vi "HaltDev.vi"(0 "输入簇":T1) -> ()   [LabVIEW 2012]
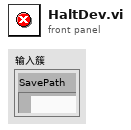
[diagram p1: front panel]
types:
  T1 = cluster{"SavePath":path, "SAVE?":bool, "connection ID":refnum<k5>}
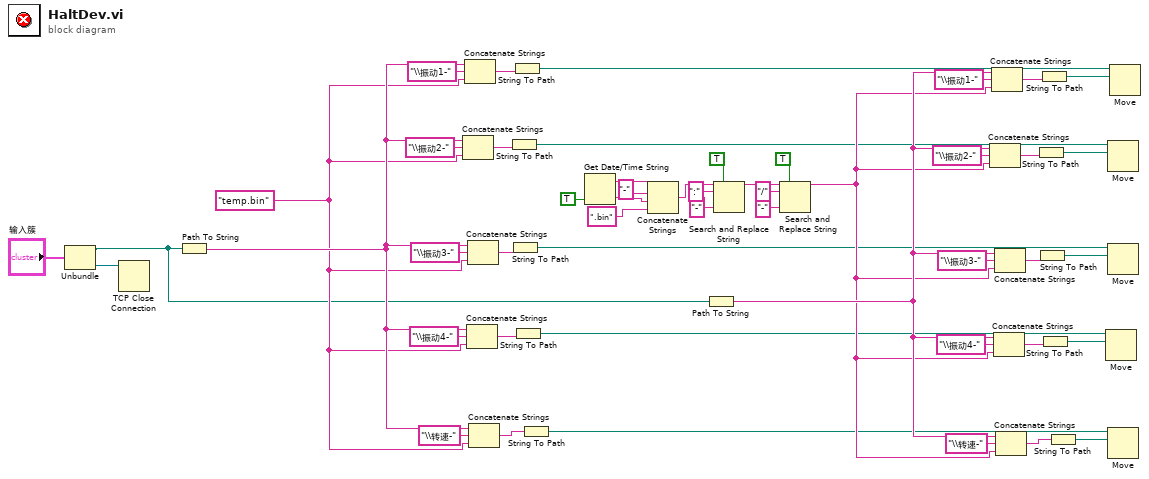
[diagram p0: block diagram]
diagram:
  w14 = "temp.bin" ("字符串")
  n1 = Unbundle("输入簇") -> ("SavePath"=w2:path, "connection ID"=w1:refnum<k5>)  [unwired: 1 out]
  n2 = TCP Close Connection(connection ID=w1) -> ()  [unwired: 2 in, 2 out]
  n3 = Path To String(path=w2) -> (string=w20:string)
  n4 = Concatenate Strings(w20, "\\振动2-" ("字符串"), w14) -> (w22:string)
  n5 = Concatenate Strings(w20, "\\振动1-" ("字符串"), w14) -> (w21:string)
  n6 = Concatenate Strings(w20, "\\振动4-" ("字符串"), w14) -> (w24:string)
  n7 = Concatenate Strings(w20, "\\振动3-" ("字符串"), w14) -> (w23:string)
  n8 = Concatenate Strings(w20, "\\转速-" ("字符串"), w14) -> (w25:string)
  n9 = String To Path(string=w22) -> (path=w11:path)
  n10 = String To Path(string=w23) -> (path=w10:path)
  n11 = String To Path(string=w21) -> (path=w13:path)
  n12 = String To Path(string=w24) -> (path=w9:path)
  n13 = String To Path(string=w25) -> (path=w8:path)
  n14 = Get Date/Time String(want seconds? (F)=TRUE ("需要秒？(F)")) -> (date string=w38:string, time string=w35:string)  [unwired: 2 in]
  n15 = Concatenate Strings(w38, "-" ("字符串"), w35, ".bin" ("字符串")) -> (w34:string)
  n16 = Path To String(path=w2) -> (string=w45:string)
  n17 = Search and Replace String(replace all?=TRUE ("替换全部？(F)"), input string=w34, search string=":" ("搜索字符串"), replace string="-" ("替换字符串(\"\")")) -> (result string=w27:string)  [unwired: 4 in, 3 out]
  n18 = Search and Replace String(replace all?=TRUE ("替换全部？(F)"), input string=w27, search string="/" ("搜索字符串"), replace string="-" ("替换字符串(\"\")")) -> (result string=w26:string)  [unwired: 4 in, 3 out]
  n19 = Concatenate Strings(w45, "\\振动2-" ("字符串"), w26) -> (w47:string)
  n20 = Concatenate Strings(w45, "\\振动1-" ("字符串"), w26) -> (w46:string)
  n21 = Concatenate Strings(w45, "\\振动4-" ("字符串"), w26) -> (w49:string)
  n22 = Concatenate Strings(w45, "\\振动3-" ("字符串"), w26) -> (w48:string)
  n23 = Concatenate Strings(w45, "\\转速-" ("字符串"), w26) -> (w50:string)
  n24 = String To Path(string=w47) -> (path=w7:path)
  n25 = String To Path(string=w48) -> (path=w6:path)
  n26 = String To Path(string=w46) -> (path=w12:path)
  n27 = String To Path(string=w49) -> (path=w5:path)
  n28 = String To Path(string=w50) -> (path=w4:path)
  n29 = Move(source path=w9, 10:w5) -> ()  [unwired: 3 in, 3 out]
  n30 = Move(source path=w11, 10:w7) -> ()  [unwired: 3 in, 3 out]
  n31 = Move(source path=w10, 10:w6) -> ()  [unwired: 3 in, 3 out]
  n32 = Move(source path=w8, 10:w4) -> ()  [unwired: 3 in, 3 out]
  n33 = Move(source path=w13, 10:w12) -> ()  [unwired: 3 in, 3 out]
